vi "get_duration.vi"(8 "error in (no error)":errorcluster, 11 "ImagingModeDL100901FlexTrajectory in":refnum<class "ImagingModeDL100901FlexTrajectory.lvclass">) -> (0 "error out":errorcluster, 1 "number of frames":i32, 2 "scan repetitions":i32, 3 "ImagingModeDL100901FlexTrajectory out":refnum<class "ImagingModeDL100901FlexTrajectory.lvclass">)   [LabVIEW 2010, in "ImagingModeDL100901FlexTrajectory.lvclass"]
uses:
  ImagingModeDL100901FlexTrajectory.lvclass
  ImagingModeDL100901FlexTrajectory.lvclass/ImagingModeDL100901FlexTrajectory.ctl
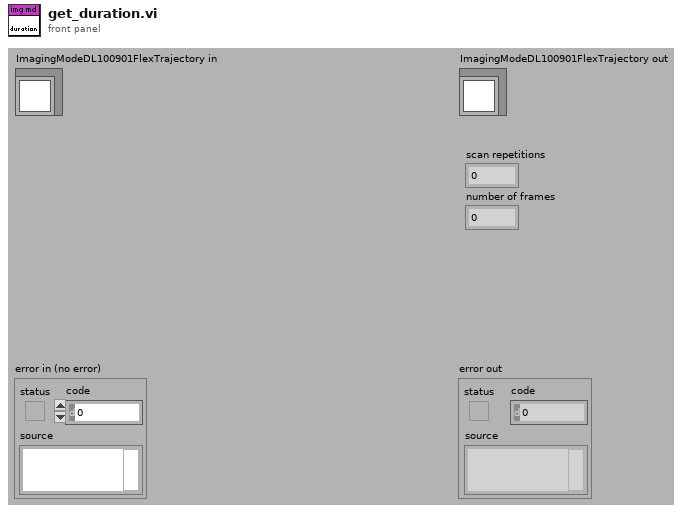
[diagram p1: front panel]
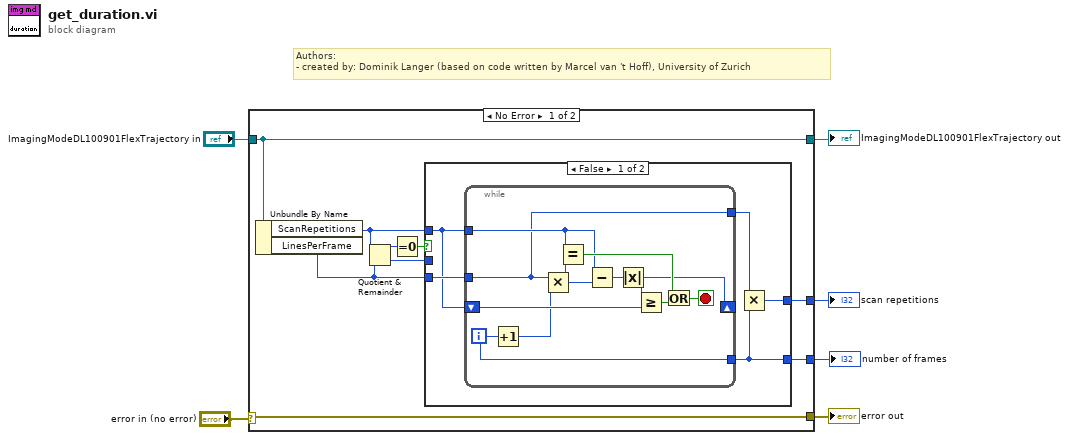
[diagram p0: block diagram]
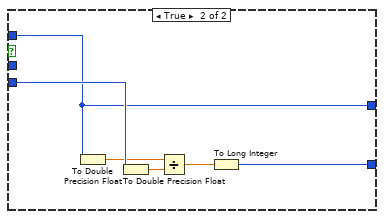
[diagram p2: hidden frame]
diagram:
  # "Authors: \n- created by: Dominik Langer (based on code written by Marcel van 't Hoff), University of Zurich"
  n1 = case shown="No Error" "error in (no error)" {
    selector: "error in (no error)" -> [w8 w38]
    tunnel: [w15 w39] -> w2
    tunnel: "ImagingModeDL100901FlexTrajectory in" -> [w15 w39]
    tunnel: [w10 _] -> w5
    tunnel: [w9 _] -> w1
    tunnel: [w8 w38] -> w4
    frame No Error {
      n2 = Unbundle By Name(w15) -> ("ScanRepetitions"=w11:i32, "LinesPerFrame"=w7:i32)
      n3 = Quotient & Remainder(x=w11, y=w7) -> (x-y*floor(x/y)=w13:i32, floor(x/y)=w12:i32)
      n4 = Equal To 0?(x=w13) -> (x = 0?=w14:bool)
      n5 = case shown="False" w14 {
        tunnel: w7 -> [w20 w36]
        tunnel: w11 -> [w19 w32]
        tunnel: [w17 w33] -> w9
        tunnel: [w16 w32] -> w10
        tunnel: w12 -> [_ _]
        frame False {
          n6 = while {
            tunnel: w20 -> [w26]
            tunnel: w19 -> [w29]
            shift-right: [w24] -> _
            shift-left: w19 -> [w25]
            tunnel: [w22] -> w17
            tunnel: [w26] -> w18
            i -> [w22]
            stop <- w23 stop-if-true
            n7 = Increment(x=w22) -> (x+1=w21:i32)
            n8 = Multiply(x=w26, y=w21) -> (x*y=w27:i32)
            n9 = Equal?(x=w29, y=w27) -> (x = y?=w31:bool)
            n10 = Subtract(x=w29, y=w27) -> (x-y=w28:i32)
            n11 = Absolute Value(x=w28) -> (abs(x)=w24:i32)
            n12 = Greater Or Equal?(x=w24, y=w25) -> (x >= y?=w30:bool)
            n13 = Or(x=w31, y=w30) -> (x .or. y?=w23:bool)
          }
          n14 = Multiply(x=w18, y=w17) -> (x*y=w16:i32)
        }
        frame True {
          n15 = To Double Precision Float(number=w32) -> (double precision float=w34:dbl)
          n16 = To Double Precision Float(number=w36) -> (double precision float=w35:dbl)
          n17 = Divide(x=w34, y=w35) -> (x/y=w37:dbl)
          n18 = To Long Integer(number=w37) -> (32bit integer=w33:i32)
        }
      }
    }
    frame Error {
    }
  }
  "error out" <- w4
  "ImagingModeDL100901FlexTrajectory out" <- w2
  "scan repetitions" <- w5
  "number of frames" <- w1
